vi "Badge Priority.vi"(11 "Code":string) -> (3 "Priority":i32)   [LabVIEW 2022 SP3, in "AoC22.lvlib"]
uses:
  AoC22.lvlib
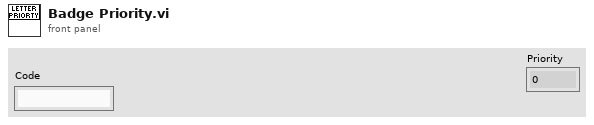
[diagram p1: front panel]
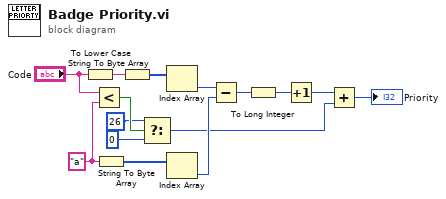
[diagram p0: block diagram]
diagram:
  w15 = "a" ("y")
  n1 = To Lower Case(string="Code") -> (all lower case string=w14:string)
  n2 = Less?(x="Code", y=w15) -> (x < y?=w9:bool)
  n3 = String To Byte Array(string=w15) -> (unsigned byte array=w12:u8[])
  n4 = String To Byte Array(string=w14) -> (unsigned byte array=w13:u8[])
  n5 = Select(t=26, s=w9, f=0) -> (s? t:f=w5:i32)
  n6 = Index Array(array=w13) -> (element=w11:u8)  [unwired: 1 in]
  n7 = Index Array(array=w12) -> (element=w10:u8)  [unwired: 1 in]
  n8 = Subtract(x=w11, y=w10) -> (x-y=w4:u8)
  n9 = To Long Integer(number=w4) -> (32bit integer=w3:i32)
  n10 = Increment(x=w3) -> (x+1=w6:i32)
  n11 = Add(x=w6, y=w5) -> (x+y=→"Priority":i32)
